vi "Module - RH_BUJAH.vi"() -> ()   [LabVIEW 2019]
uses:
  Control/State - eFGV.ctl
panel:
  out "Site Name":string="RH BUJAH (34.58 kWp)"
  out "STP-04-STATUS":bool
  out "STP-04-B-IDC":dbl caption="B.Idc" format="%.1f A"
  out "STP-04-B-VDC":dbl caption="B.Vdc" format="%.0f V"
  out "STP-04-A-IDC":dbl caption="A.Idc" format="%.1f A"
  out "STP-04-A-VDC":dbl caption="A.Vdc" format="%.0f V"
  out "STP-04-PAC":dbl caption="Pac" format="%#_g W"
  out "BANK-04-TEMP":dbl caption="T_bat" format="%#_g °C"
  out "BANK-04-IDC":dbl caption="I_bat" format="%.2f A"
  out "BANK-04-VDC":dbl caption="V_bat" format="%.1f V"
  out "BANK-04-SOC":dbl caption="SOC" format="%#_g %"
  out "BANK-03-TEMP":dbl caption="T_bat" format="%#_g °C"
  out "BANK-03-IDC":dbl caption="I_bat" format="%.2f A"
  out "BANK-03-VDC":dbl caption="V_bat" format="%.1f V"
  out "BANK-03-SOC":dbl caption="SOC" format="%#_g %"
  out "SI-M-02-STATUS":bool
  out "SI-M-02-FREQ":dbl caption="FREQ" format="%.0f Hz"
  out "SI-M-02-L3":dbl caption="L3" format="%.0f V"
  out "SI-M-02-L2":dbl caption="L2" format="%.0f V"
  out "SI-M-02-L1":dbl caption="L1" format="%.0f V"
  out "SI-M-02-PAC":dbl caption="Pac" format="%.0f W"
  out "STP-03-STATUS":bool
  out "STP-03-B-IDC":dbl caption="B.Idc" format="%.1f A"
  out "STP-03-B-VDC":dbl caption="B.Vdc" format="%.0f V"
  out "STP-03-A-IDC":dbl caption="A.Idc" format="%.1f A"
  out "STP-03-A-VDC":dbl caption="A.Vdc" format="%.0f V"
  out "STP-03-PAC":dbl caption="Pac" format="%#_g W"
  out "PM-01-STATUS":bool
  out "SI-M-01-STATUS":bool
  out "STP-02-STATUS":bool
  out "STP-01-STATUS":bool
  out "BANK-02-TEMP":dbl caption="T_bat" format="%#_g °C"
  out "BANK-02-IDC":dbl caption="I_bat" format="%.2f A"
  out "BANK-02-VDC":dbl caption="V_bat" format="%.1f V"
  out "BANK-02-SOC":dbl caption="SOC" format="%#_g %"
  out "STP-02-B-IDC":dbl caption="B.Idc" format="%.1f A"
  out "STP-02-B-VDC":dbl caption="B.Vdc" format="%.0f V"
  out "STP-02-A-IDC":dbl caption="A.Idc" format="%.1f A"
  out "STP-02-A-VDC":dbl caption="A.Vdc" format="%.0f V"
  out "STP-02-PAC":dbl caption="Pac" format="%#_g W"
  out "PM-01-FREQ":dbl caption="Freq" format="%.0f Hz"
  out "PM-01-IAC":dbl caption="Iac" format="%.0f A"
  out "PM-01-VAC":dbl caption="Vac" format="%.0f V"
  out "PM-01-PAC":dbl caption="Pac" format="%.0f W"
  out "SI-M-01-FREQ":dbl caption="FREQ" format="%.0f Hz"
  out "SI-M-01-L3":dbl caption="L3" format="%.0f V"
  out "SI-M-01-L2":dbl caption="L2" format="%.0f V"
  out "SI-M-01-L1":dbl caption="L1" format="%.0f V"
  out "SI-M-01-PAC":dbl caption="Pac" format="%.0f W"
  out "BANK-01-TEMP":dbl caption="T_bat" format="%#_g °C"
  out "BANK-01-IDC":dbl caption="I_bat" format="%.2f A"
  out "BANK-01-VDC":dbl caption="V_bat" format="%.1f V"
  out "BANK-01-SOC":dbl caption="SOC" format="%#_g %"
  out "STP-01-B-IDC":dbl caption="B.Idc" format="%.1f A"
  out "STP-01-B-VDC":dbl caption="B.Vdc" format="%.0f V"
  out "STP-01-A-IDC":dbl caption="A.Idc" format="%.1f A"
  out "STP-01-A-VDC":dbl caption="A.Vdc" format="%.0f V"
  out "STP-01-PAC":dbl caption="Pac" format="%.0f W"
  # "BANK-1"
  # "BANK-2"
  # "STP-02"
  # "BANK-1"
  # "BANK-2"
  # "STP-01"
  # "SI-M-02"
  # "SI-M-01"
  # "STP-03"
  # "STP-04"
  # "PM-01"
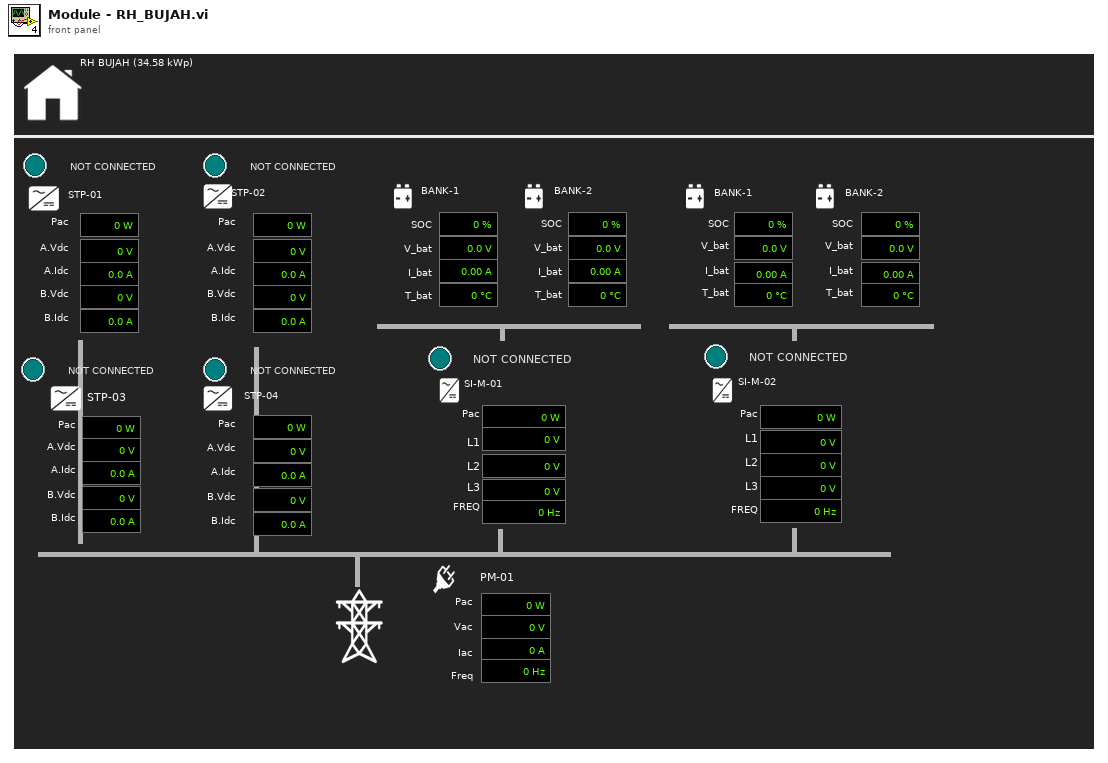
[diagram p1: front panel]
types:
  T1 = typedef "State - eFGV.ctl" = enum16{"Init", "Read", "Write", "Close"}
  T2 = typedef "Device Name.ctl" = enum16{"SB-01", "SB-02", "SB-03", "SB-04", "STP-01", "STP-02", "STP-03", "STP-04", "BANK-01", "BANK-02", "BANK-03", "BANK-04", "SI-M-01", "SI-M-02", "SI-M-03", "SI-M-04", "PM-01", "PM-02", "PM-03", "PM-04"}
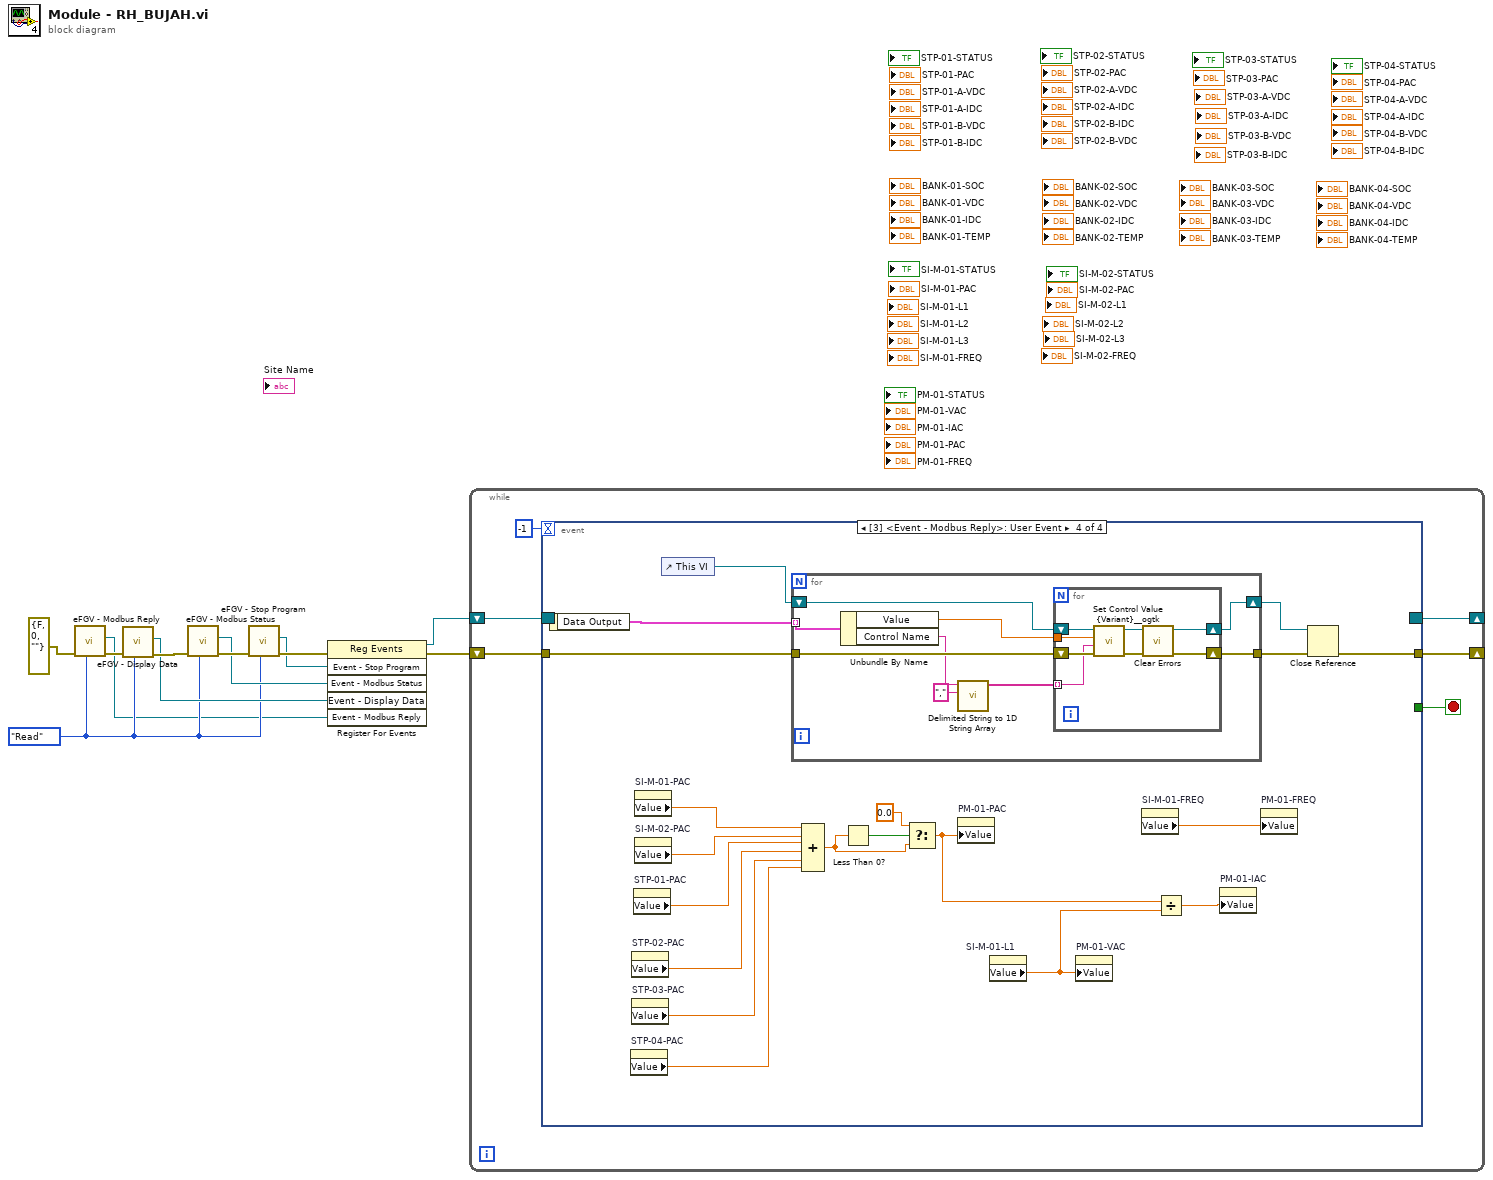
[diagram p0: block diagram]
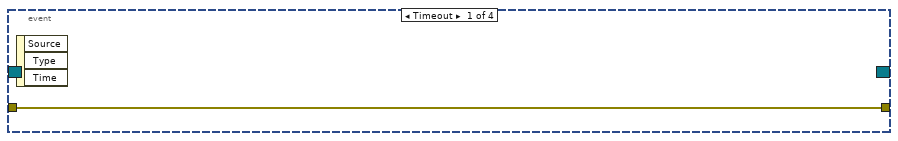
[diagram p2: hidden frame]
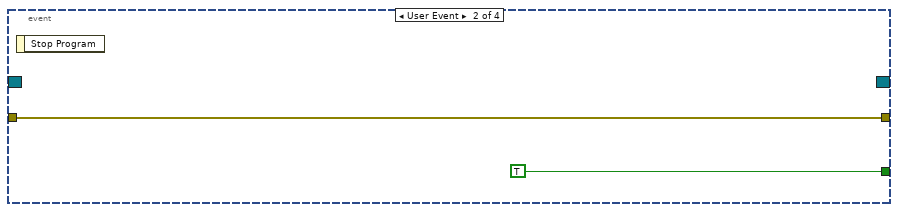
[diagram p3: hidden frame]
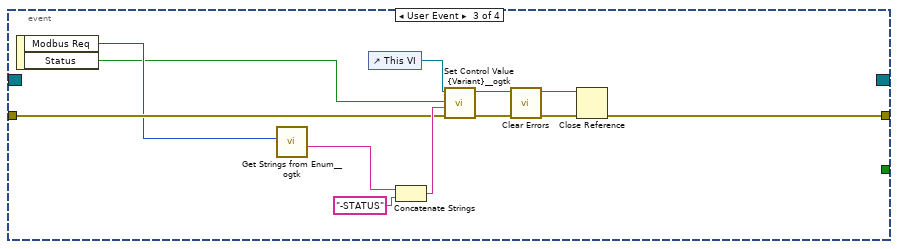
[diagram p4: hidden frame]
diagram:
  w2 = State_-_eFGV."Read" ("State - eFGV")
  n1 = call "eFGV - Modbus Reply.vi"("State - eFGV"=w2, "error in (no error)"=errorcluster {"status"=FALSE, "code"=0, "source"=""}) -> ("error out"=w3:errorcluster, "Event - Modbus Reply"=w1:refnum<user-event>)  [unwired: 8 in]
  n2 = call "eFGV - Display Data.vi"("State - eFGV"=w2, "error in (no error)"=w3) -> ("error out"=w7:errorcluster, "Event - Display Data"=w6:refnum<user-event>)  [unwired: 8 in]
  n3 = call "eFGV - Modbus Status.vi"("State - eFGV"=w2, "error in (no error)"=w7) -> ("error out"=w9:errorcluster, "Event - Modbus Status"=w8:refnum<user-event>)  [unwired: 8 in]
  n4 = call "eFGV - Stop Program.vi"("State - eFGV"=w2, "error in (no error)"=w9) -> ("error out"=w12:errorcluster, "Event - Stop Program"=w11:refnum<user-event>)  [unwired: 8 in]
  n5 = register-events(error in=w12, w11, w8, w6, w1) -> (reference out=w10:refnum<event-registration>, error out=w5:errorcluster)  [unwired: 1 in]
  n6 = while {
    shift-right: [w17] -> _
    shift-left: w10 -> [w18]
    shift-right: [w14] -> _
    shift-left: w5 -> [w13]
    stop <- w16 stop-if-true
    n7 = event shown="[3] <Event - Modbus Reply>: User Event" {
      selector: w18 -> [_ _ _ _]
      dyn-events: [_ _ _ _] -> w17
      timeout: -1 -> [_ _ _ _]
      tunnel: w13 -> [w19 w20 w26 w47]
      tunnel: [_ TRUE _ _] -> w16
      tunnel: [w19 w20 w23 w49] -> w14
      event Timeout {
        n8 = event-data() -> ()  [unwired: 1 in, 3 out]
      }
      event User Event {
        n9 = event-data() -> ()  [unwired: 1 in, 1 out]
      }
      event User Event {
        n10 = event-data() -> ("Modbus Req"=w25:T2, "Status"=w24:bool)  [unwired: 1 in]
        n11 = call "Get Strings from Enum__ogtk.vi"("Enum"=w25) -> ("String Value"=w28:string)  [unwired: 7 in, 3 out]
        n12 = control-ref of="This VI"() -> (w32:refnum<vi>)
        n13 = Concatenate Strings(w28, "-STATUS" ("string")) -> (w31:string)
        n14 = call "Set Control Value {Variant}__ogtk.vi"("error in (no error)"=w26, "Control Name (\"\": use variant name)"=w31, "Value"=w24, "VI Refnum"=w32) -> ("error out"=w30:errorcluster, "VI Refnum dup"=w29:refnum<vi>)  [unwired: 6 in]
        n15 = call <vilib>:"Clear Errors.vi"("error in (no error)"=w30) -> ("error out"=w22:errorcluster)  [unwired: 5 in, 1 out]
        n16 = Close Reference(reference=w29, error in (no error)=w22) -> (error out=w23:errorcluster)
      }
      event User Event {
        n17 = event-data() -> ("Data Output"=w48:cluster{"Control Name":string, "Value":dbl}[])  [unwired: 1 in]
        n18 = property on="STP-04-PAC" class="DigNum (strict)"() -> ("Value"=w34:dbl)  [unwired: 2 in, 2 out]
        n19 = property on="STP-02-PAC" class="DigNum (strict)"() -> ("Value"=w36:dbl)  [unwired: 2 in, 2 out]
        n20 = property on="STP-03-PAC" class="DigNum (strict)"() -> ("Value"=w35:dbl)  [unwired: 2 in, 2 out]
        n21 = property on="STP-01-PAC" class="DigNum (strict)"() -> ("Value"=w43:dbl)  [unwired: 2 in, 2 out]
        n22 = property on="SI-M-01-PAC" class="DigNum (strict)"() -> ("Value"=w45:dbl)  [unwired: 2 in, 2 out]
        n23 = property on="SI-M-02-PAC" class="DigNum (strict)"() -> ("Value"=w44:dbl)  [unwired: 2 in, 2 out]
        n24 = control-ref of="This VI"() -> (w33:refnum<vi>)
        n25 = for {
          tunnel: w47 -> [w60]
          tunnel: [w59] -> w51
          tunnel: w48 -> [w57] mode=indexing
          shift-right: [w58] -> w50
          shift-left: w33 -> [w52]
          n26 = Unbundle By Name(w57) -> ("Value"=w56:dbl, "Control Name"=w55:string)
          n27 = call <vilib>:"Delimited String to 1D String Array.vi"("delimiter"=",", "delimited string"=w55) -> ("string array"=w53:string[])  [unwired: 9 in]
          n28 = for {
            tunnel: w56 -> [w63]
            shift-right: [w64] -> w58
            shift-left: w52 -> [w67]
            shift-right: [w61] -> w59
            shift-left: w60 -> [w66]
            tunnel: w53 -> [w62] mode=indexing
            n29 = call "Set Control Value {Variant}__ogtk.vi"("error in (no error)"=w66, "Control Name (\"\": use variant name)"=w62, "Value"=w63, "VI Refnum"=w67) -> ("error out"=w65:errorcluster, "VI Refnum dup"=w64:refnum<vi>)  [unwired: 6 in]
            n30 = call <vilib>:"Clear Errors.vi"("error in (no error)"=w65) -> ("error out"=w61:errorcluster)  [unwired: 5 in, 1 out]
          }
        }
        n31 = Compound Arithmetic op=ADD(w45, w44, w43, w36, w35, w34) -> (w41:dbl)
        n32 = Less Than 0?(x=w41) -> (x < 0?=w42:bool)
        n33 = Select(t=0.0, s=w42, f=w41) -> (s? t:f=w38:dbl)
        n34 = property on="PM-01-PAC" class="DigNum (strict)"("Value"=w38) -> ()  [unwired: 2 in, 2 out]
        n35 = property on="SI-M-01-L1" class="DigNum (strict)"() -> ("Value"=w37:dbl)  [unwired: 2 in, 2 out]
        n36 = property on="PM-01-VAC" class="DigNum (strict)"("Value"=w37) -> ()  [unwired: 2 in, 2 out]
        n37 = property on="SI-M-01-FREQ" class="DigNum (strict)"() -> ("Value"=w46:dbl)  [unwired: 2 in, 2 out]
        n38 = Divide(x=w38, y=w37) -> (x/y=w39:dbl)
        n39 = property on="PM-01-IAC" class="DigNum (strict)"("Value"=w39) -> ()  [unwired: 2 in, 2 out]
        n40 = property on="PM-01-FREQ" class="DigNum (strict)"("Value"=w46) -> ()  [unwired: 2 in, 2 out]
        n41 = Close Reference(reference=w50, error in (no error)=w51) -> (error out=w49:errorcluster)
      }
    }
  }
